vi "Initialize Folder Structure.vi"(8 "error in (no error)":errorcluster, 11 "Project in":refnum<class "Project.lvclass">) -> (0 "error out":errorcluster, 3 "Project out":refnum<class "Project.lvclass">)   [LabVIEW 2015, in "Project.lvclass"]
uses:
  Project.lvclass
  Project.lvclass/Project.ctl
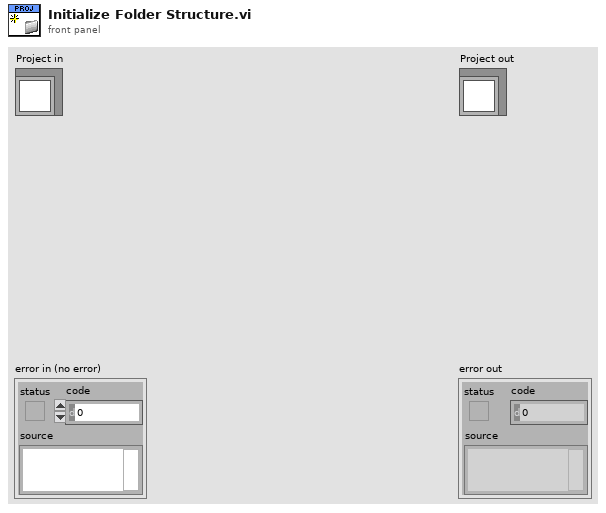
[diagram p1: front panel]
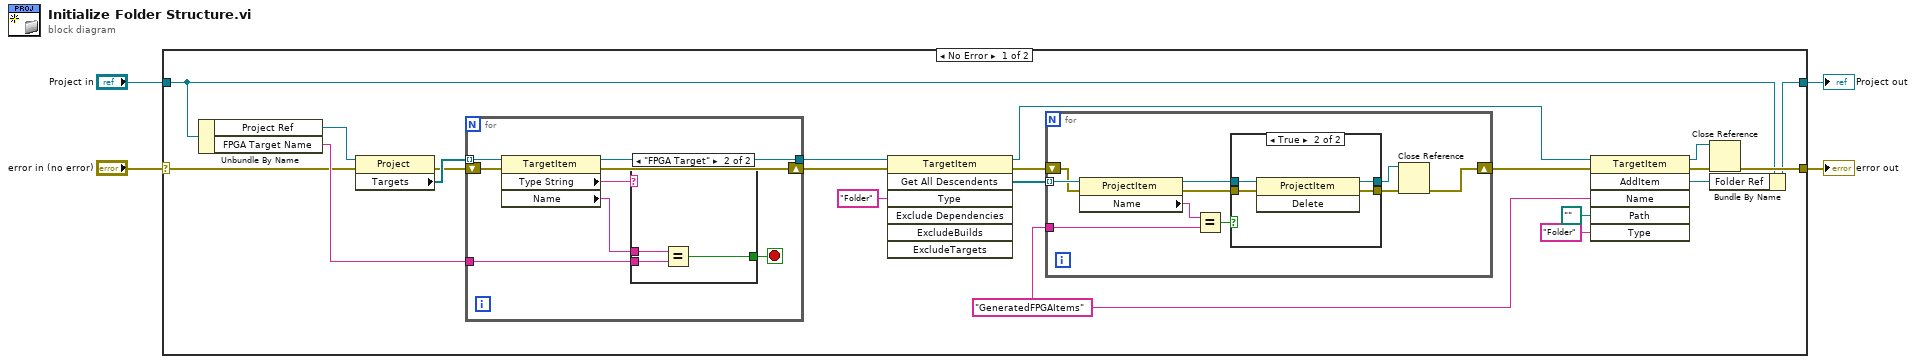
[diagram p0: block diagram]
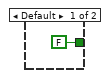
[diagram p2: hidden frame]
diagram:
  n1 = case shown="No Error" "error in (no error)" {
    selector: "error in (no error)" -> [w5 w55]
    tunnel: [w11 w55] -> w3
    tunnel: [w7 w54] -> w1
    tunnel: "Project in" -> [w8 w54]
    frame No Error {
      w14 = "GeneratedFPGAItems" ("Name")
      n2 = Unbundle By Name(w8) -> ("Project Ref"=w6:refnum<vi>, "FPGA Target Name"=w10:string)
      n3 = property class="Project"(reference=w6, error in=w5) -> (error out=w18:errorcluster, "Targets"=w19:refnum<vi>[])  [unwired: 1 out]
      n4 = for {
        tunnel: w19 -> [w33] mode=indexing
        tunnel: w10 -> [w32]
        shift-right: [w29] -> w17
        shift-left: w18 -> [w30]
        tunnel: [w28] -> w16
        stop <- w27 stop-if-true
        n5 = property class="TargetItem"(reference=w33, error in=w30) -> (reference out=w28:refnum<vi>, error out=w29:errorcluster, "Type String"=w26:string, "Name"=w31:string)
        n6 = case shown="\"FPGA Target\"" w26 {
          tunnel: w32 -> [_ w37]
          tunnel: w31 -> [_ w36]
          tunnel: [FALSE w35] -> w27
          frame Default {
          }
          frame "FPGA Target" {
            n7 = Equal?(x=w36, y=w37) -> (x = y?=w35:bool)
          }
        }
      }
      n8 = invoke class="TargetItem" method="Get All Descendents"(reference=w16, error in=w17, "Type"="Folder") -> (reference out=w15:refnum<vi>, error out=w20:errorcluster, "All Descendents"=w21:refnum<vi>[])  [unwired: 4 in, 4 out]
      n9 = for {
        tunnel: w21 -> [w47] mode=indexing
        shift-right: [w38] -> w24
        shift-left: w20 -> [w46]
        tunnel: w14 -> [w44]
        n10 = property class="ProjectItem"(reference=w47, error in=w46) -> (reference out=w43:refnum<vi>, error out=w42:errorcluster, "Name"=w45:string)
        n11 = Equal?(x=w45, y=w44) -> (x = y?=w41:bool)
        n12 = case shown="True" w41 {
          tunnel: w43 -> [w48 w53]
          tunnel: w42 -> [w49 w52]
          tunnel: [w49 w51] -> w39
          tunnel: [w48 w50] -> w40
          frame False {
          }
          frame True {
            n13 = invoke class="ProjectItem" method="Delete"(reference=w53, error in=w52) -> (reference out=w50:refnum<vi>, error out=w51:errorcluster)  [unwired: 1 in, 1 out]
          }
        }
        n14 = Close Reference(reference=w40, error in (no error)=w39) -> (error out=w38:errorcluster)
      }
      n15 = invoke class="TargetItem" method="AddItem"(reference=w15, error in=w24, "Name"=w14, "Path"=path "", "Type"="Folder") -> (reference out=w13:refnum<vi>, error out=w12:errorcluster, "AddItem"=w9:refnum<vi>)  [unwired: 1 in, 3 out]
      n16 = Close Reference(reference=w13, error in (no error)=w12) -> (error out=w11:errorcluster)
      n17 = Bundle By Name(cluster=w8, "Folder Ref"=w9) -> (w7:refnum<class "Project.lvclass">)
    }
    frame Error {
    }
  }
  "error out" <- w3
  "Project out" <- w1
